vi "Test Template Creation.vi"() -> ()   [LabVIEW 2020, in "Template Tool.lvlib"]
uses:
  Template Tool.lvlib
panel:
  in  "custom device name":string="My New Comms"
  out "error out":errorcluster
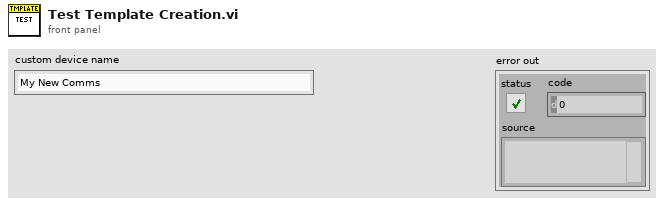
[diagram p1: front panel]
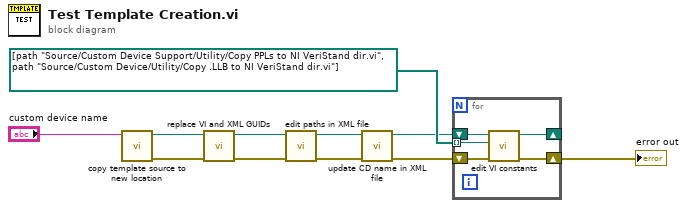
[diagram p0: block diagram]
diagram:
  n1 = call "copy template source to new location.vi"("custom device name"="custom device name") -> ("error out"=w10:errorcluster, "custom device path out"=w11:path)  [unwired: 9 in]
  n2 = call "replace VI and XML GUIDs.vi"("error in"=w10, "custom device path"=w11) -> ("error out"=w7:errorcluster, "custom device path out"=w8:path)  [unwired: 8 in]
  n3 = call "edit paths in XML file.vi"("error in"=w7, "custom device path"=w8) -> ("error out"=w2:errorcluster, "custom device path out"=w4:path)  [unwired: 8 in]
  n4 = call "update CD name in XML file.vi"("error in"=w2, "custom device path"=w4) -> ("error out"=w1:errorcluster, "custom device path out"=w3:path)  [unwired: 8 in]
  n5 = for {
    shift-right: [w14] -> w5
    shift-left: w1 -> [w15]
    tunnel: path[] [path "Source/Custom Device Support/Utility/Copy PPLs to NI VeriStand dir.vi", path "Source/Custom Device/Utility/Copy .LLB to NI VeriStand dir.vi"] -> [w13] mode=indexing
    shift-right: [w12] -> _
    shift-left: w3 -> [w16]
    n6 = call "edit VI constants.vi"("error in"=w15, "relative path of VI to edit"=w13, "custom device path"=w16) -> ("error out"=w14:errorcluster, "custom device path out"=w12:path)  [unwired: 7 in]
  }
  "error out" <- w5
